vi "Threshold_2D_Array.vi"(0 "2D Array IN":sgl[][](array[numeric]), 7 "Upper Limit":dbl, 11 "Lower Limit":dbl) -> (8 "Threshold Array Out":dbl[](array[numeric]))   [LabVIEW 2016]
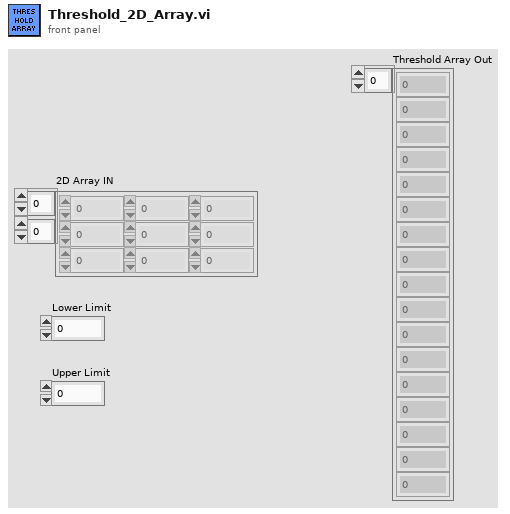
[diagram p1: front panel]
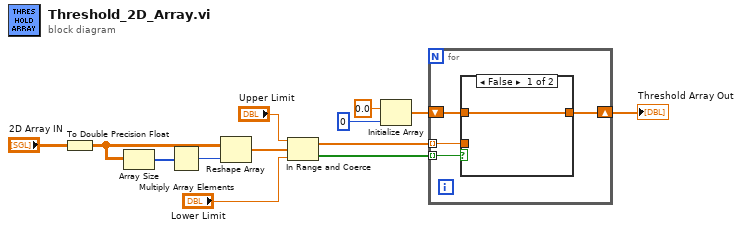
[diagram p0: block diagram]
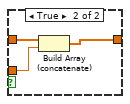
[diagram p2: hidden frame]
diagram:
  n1 = To Double Precision Float(number="2D Array IN") -> (double precision float=w13:dbl[][])
  n2 = Array Size(array=w13) -> (size(s)=w11:i32[])
  n3 = Multiply Array Elements(1:w11) -> (0:w12:i32)
  n4 = Reshape Array(w13, w12) -> (w7:dbl[])
  n5 = In Range and Coerce(upper limit="Upper Limit", x=w7, lower limit="Lower Limit") -> (coerced(x)=w3:dbl[], In Range?=w2:bool[])
  n6 = Initialize Array(0.0 ("element"), 0 ("dimension size")) -> (w4:dbl[])
  n7 = for {
    shift-right: [w14] -> w1
    shift-left: w4 -> [w17]
    tunnel: w3 -> [w15] mode=indexing
    tunnel: w2 -> [w16] mode=indexing
    n8 = case shown="False" w16 {
      tunnel: w17 -> [w18 w21]
      tunnel: w15 -> [_ w20]
      tunnel: [w18 w19] -> w14
      frame False {
      }
      frame True {
        n9 = Build Array (concatenate)(w21, w20) -> (w19:dbl[])
      }
    }
  }
  "Threshold Array Out" <- w1
